vi "User Access Level FGV.vi"(7 "Use Level Cmd":T1, 8 "Error In":errorcluster, 10 "User Name":string) -> (0 "Error Out":errorcluster, 1 "User Level":string)   [LabVIEW 2018]
doc: "This FGV holds the Access Level for the user currently logged in. It executes the following methods:\n\n1. <B>Read User Access Level File:</B> Reads a tab-delimited text file containing User Names and corresponding Access Levels.\n2. <B>Set Current Access Level:</B> Sets the Access level for the User Name input.\n3. <B>Get Current Access Level:</B> Returns the Access level for the current User."
uses:
  User Level Cmd.ctl
  <vilib>/Utility/file.llb/Read Delimited Spreadsheet (string).vi
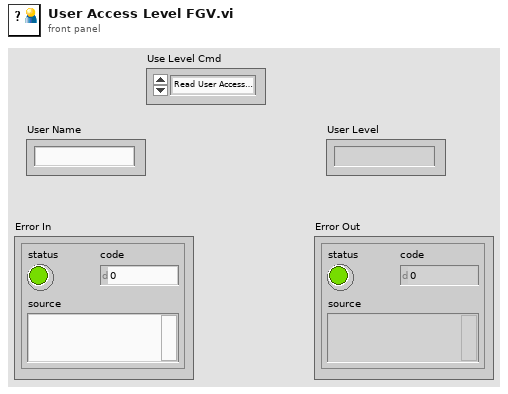
[diagram p1: front panel]
types:
  T1 = typedef "User Level Cmd.ctl" = enum16{"Read User Access Level File", "Set Current User", "Get User Access Level"}
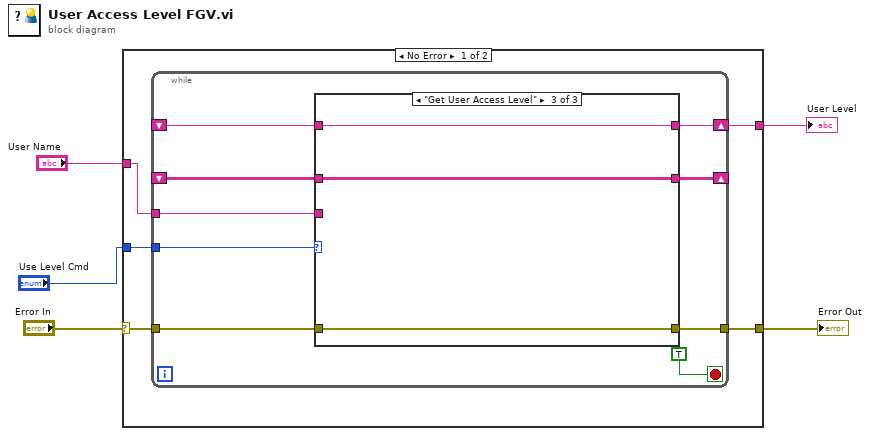
[diagram p0: block diagram]
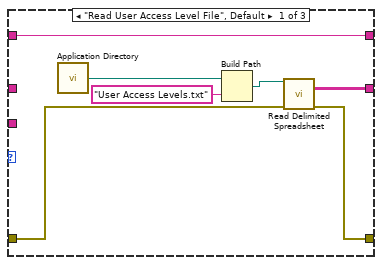
[diagram p2: hidden frame]
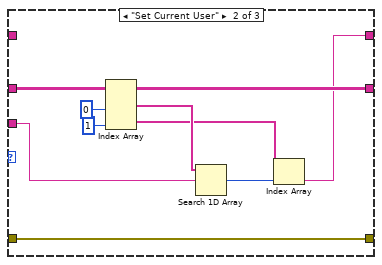
[diagram p3: hidden frame]
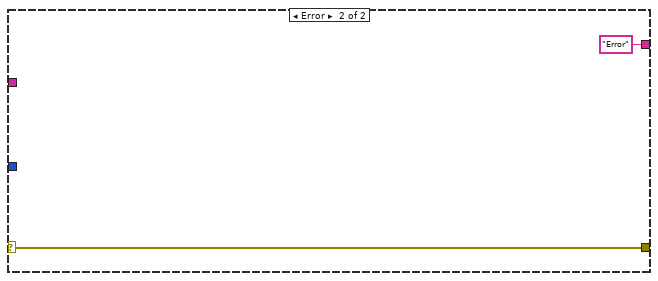
[diagram p4: hidden frame]
diagram:
  n1 = case shown="No Error" "Error In" {
    selector: "Error In" -> [w8 w40]
    tunnel: "Use Level Cmd" -> [w10 _]
    tunnel: "User Name" -> [w7 _]
    tunnel: [w9 w40] -> w2
    tunnel: [w6 "Error" ("String")] -> w1
    frame No Error {
      n2 = while {
        tunnel: w10 -> [w18]
        tunnel: [w17] -> w9
        tunnel: w8 -> [w16]
        shift-right: [w15] -> _
        shift-left: _ -> [w14]
        shift-right: [w12] -> w6
        shift-left: _ -> [w11]
        tunnel: w7 -> [w13]
        stop <- TRUE stop-if-true
        n3 = case shown="\"Get User Access Level\"" w18 {
          tunnel: [w22 w35 w38] -> w17
          tunnel: w16 -> [w23 w35 w38]
          tunnel: [w21 w34 w37] -> w15
          tunnel: w14 -> [_ w34 w37]
          tunnel: w13 -> [_ w30 _]
          tunnel: [w20 w27 w36] -> w12
          tunnel: w11 -> [w20 _ w36]
          frame "Read User Access Level File", Default {
            n4 = call <vilib>:"Application Directory.vi"() -> ("Application Directory"=w26:path)
            n5 = Build Path(base path=w26, name or relative path="User Access Levels.txt") -> (appended path=w24:path)
            n6 = call-poly <vilib>:"Read Delimited Spreadsheet.vi"("file path (dialog if empty)"=w24, "error in (no error)"=w23) -> ("all rows"=w21:string[][], "error out"=w22:errorcluster)  [unwired: 8 in, 4 out]
          }
          frame "Set Current User" {
            n7 = Index Array(array=w34, index (col) #1=0 ("disabled index (col)"), index (col) #2=1 ("index (col)")) -> (element #1=w31:string[], element #2=w29:string[])  [unwired: 2 in]
            n8 = Search 1D Array(1D array=w31, element=w30) -> (index of element=w28:i32)  [unwired: 1 in]
            n9 = Index Array(array=w29, index=w28) -> (element=w27:string)
          }
          frame "Get User Access Level" {
          }
        }
      }
    }
    frame Error {
    }
  }
  "User Level" <- w1
  "Error Out" <- w2
